vi "3.5.vi"() -> ()   [LabVIEW 2017]
panel:
  out "Y":dbl
  in  "X":dbl
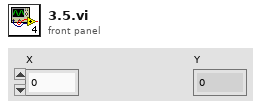
[diagram p1: front panel]
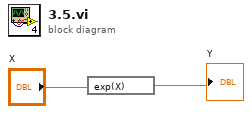
[diagram p0: block diagram]
diagram:
  n1 = expression code="exp(X)"("X") -> (→"Y":dbl)
